vi "LLB Pre-Build CHM Build.vi"(6 "Top Level/Always Included VIs":path[](array[path]), 7 "Main Destination Path":path, 9 "Target Name":string, 10 "Build Specification Name":string, 11 "Project Path":path) -> (0 "error out":errorcluster)   [LabVIEW 2020]
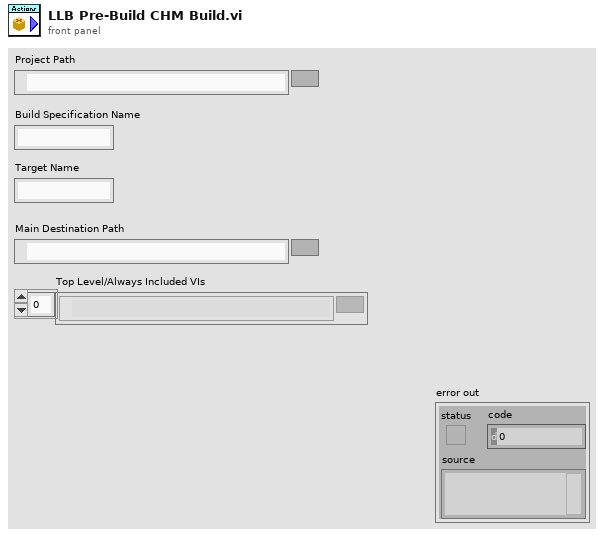
[diagram p1: front panel]
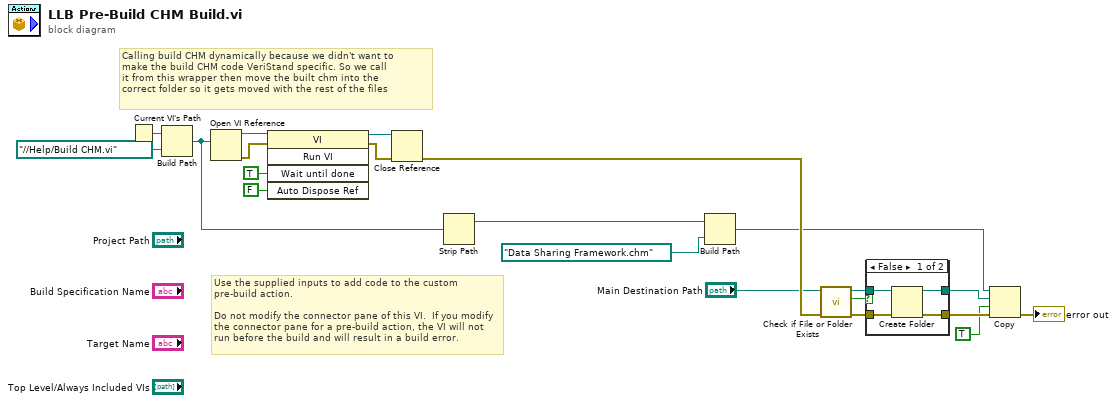
[diagram p0: block diagram]
diagram:
  # "Calling build CHM dynamically because we didn't want to \nmake the build CHM code VeriStand specific. So we call\nit from this wrapper then move the built chm into the\ncorrect folder so it gets moved with the rest of the files"
  # "Use the supplied inputs to add code to the custom pre-build action.\n\nDo not modify the connector pane of this VI.  If you modify the connector pane for a pre-build action, the VI will not run before the build and will result in a build error."
  n1 = Current VI's Path() -> (path=w21:path)
  n2 = Build Path(base path=w21, name or relative path=path "../../Help/Build CHM.vi") -> (appended path=w13:path)
  n3 = Open VI Reference(vi path=w13) -> (vi reference=w19:refnum<vi>, error out=w18:errorcluster)  [unwired: 5 in]
  n4 = invoke class="VI" method="Run VI"(reference=w19, error in=w18, "Wait until done"=TRUE ("Wait Until Done"), "Auto Dispose Ref"=FALSE ("Auto Dispose Reference")) -> (reference out=w15:refnum<vi>, error out=w14:errorcluster)  [unwired: 1 in, 3 out]
  n5 = Close Reference(reference=w15, error in (no error)=w14) -> (error out=w12:errorcluster)
  n6 = Strip Path(path=w13) -> (stripped path=w3:path)  [unwired: 1 out]
  n7 = Build Path(base path=w3, name or relative path=path "Data Sharing Framework.chm" ("stripped path")) -> (appended path=w5:path)
  n8 = call <vilib>:"Check if File or Folder Exists.vi"("error in (no error)"=w12, "path"="Main Destination Path") -> ("error out"=w9:errorcluster, "file or folder exists?"=w11:bool, "dup path"=w10:path)  [unwired: 7 in]
  n9 = case shown="False" w11 {
    tunnel: w10 -> [w24 w27]
    tunnel: w9 -> [w25 w26]
    tunnel: [w23 w27] -> w7
    tunnel: [w22 w26] -> w8
    frame False {
      n10 = Create Folder(path (use dialog)=w24, error in=w25) -> (created path=w23:path, error out=w22:errorcluster)  [unwired: 1 in, 1 out]
    }
    frame True {
    }
  }
  n11 = Copy(8:w8, 9:TRUE ("overwrite (F)"), 10:w7, 11:w5) -> (0:→"error out":errorcluster)  [unwired: 1 in, 2 out]
